vi "ReactionWheel RT - autostarted.vi"() -> ()   [LabVIEW 2021]
uses:
  <vilib>/Platform/TimedLoop/XDataNode/timing_clust.ctl
  <vilib>/Platform/TimedLoop/XDataNode/nitl_modes.ctl
  <vilib>/Platform/TimedLoop/XDataNode/wakeup.ctl
  <vilib>/myRIO/Instrument Drivers/Onboard IO/UART/typedef/VISA Configuration.ctl
  <vilib>/myRIO/Instrument Drivers/Onboard IO/DIO/typedefs/DIO Reference.ctl
  <vilib>/myRIO/Common/Instrument Driver Framework/Utilities/typedefs/myRIO Generic Hardware Reference.ctl
  <vilib>/myRIO/Common/Instrument Driver Framework/Utilities/typedefs/Hardware Version Enum.ctl
  <vilib>/myRIO/Common/Instrument Driver Framework/Utilities/typedefs/myRIO v1.0 Reference.ctl
  <vilib>/myRIO/Common/Instrument Driver Framework/Utilities/typedefs/Generic FPGA Reference.ctl
  <vilib>/myRIO/Common/Instrument Driver Framework/myRIO v1.0/DIO/typedefs/DIO Channels List.ctl
  <vilib>/myRIO/Common/Instrument Driver Framework/myRIO v1.0/DIO/typedefs/DIO Channels Enum.ctl
  <vilib>/userdefined/High Color/nirio_resource_hc.ctl
  <vilib>/myRIO/Instrument Drivers/Onboard IO/PWM/typedefs/PWM Reference.ctl
  <vilib>/myRIO/Common/Instrument Driver Framework/myRIO v1.0/PWM/typedefs/PWM Channels Enum.ctl
  <vilib>/myRIO/Instrument Drivers/Onboard IO/PWM/typedefs/PWM Configuration.ctl
  <vilib>/myRIO/Common/Instrument Driver Framework/Utilities/vis/Is FPGA Ref Available.vi
  <vilib>/myRIO/Common/Instrument Driver Framework/myRIO v1.0/PWM/vis/myRIO v1.1 Open PWM.vi
  <vilib>/myRIO/Instrument Drivers/Onboard IO/PWM/vis/Set Duty Cycle and Frequency.vi
  <vilib>/myRIO/Common/Instrument Driver Framework/myRIO v1.0/DIO/vis/myRIO v1.1 Open DIO.vi
  <vilib>/myRIO/Instrument Drivers/Onboard IO/DIO/vis/Write.vi
  <vilib>/myRIO/Common/Instrument Driver Framework/Utilities/vis/Validate Channels.vi
  <vilib>/myRIO/Common/Instrument Driver Framework/myRIO v1.0/PWM/vis/myRIO v1.0 Reserve PWM.vi
  <vilib>/myRIO/Common/Instrument Driver Framework/myRIO v1.0/DIO/vis/myRIO v1.0 Reserve DIO.vi
  <vilib>/myRIO/Common/Instrument Driver Framework/myRIO v1.0/PWM/vis/myRIO v1.0 Build MUX Configuration PWM.vi
  <vilib>/myRIO/Common/Instrument Driver Framework/myRIO v1.0/Resource Manager/vis/myRIO v1.0 Reserve Channel List.vi
  <vilib>/myRIO/Common/Instrument Driver Framework/myRIO v1.0/DIO/vis/myRIO v1.0 Build MUX Configuration DIO.vi
  <vilib>/myRIO/Common/Instrument Driver Framework/myRIO v1.0/Resource Manager/vis/myRIO v1.0 Create Configuration List.vi
  <vilib>/myRIO/Common/Instrument Driver Framework/myRIO v1.0/Resource Manager/vis/myRIO v1.0 Reserve Channel.vi
  <vilib>/myRIO/Common/Instrument Driver Framework/myRIO v1.0/Resource Manager/vis/myRIO v1.0 Unreserve Channel.vi
  <vilib>/myRIO/Common/Instrument Driver Framework/myRIO v1.0/Resource Manager/vis/myRIO v1.0 Build Mutex Name.vi
  <vilib>/Instr/_visa.llb/VISA Configure Serial Port (Instr).vi
  <vilib>/Utility/VariantDataType/GetNumericInfo.vi
  <vilib>/Utility/error.llb/Error Cluster From Error Code.vi
  <vilib>/myRIO/Common/Instrument Driver Framework/myRIO v1.0/myRIO v1.1 Open.vi
  <vilib>/myRIO/Common/Instrument Driver Framework/Utilities/vis/IO Manager.vi
  <vilib>/myRIO/Common/Instrument Driver Framework/Utilities/vis/Configuration Manager.vi
  <vilib>/myRIO/Common/Instrument Driver Framework/myRIO v1.0/Resource Manager/vis/myRIO v1.0 Configure IO.vi
  <vilib>/myRIO/Common/Instrument Driver Framework/myRIO v1.0/myRIO v1.0 Close.vi
  <vilib>/myRIO/Common/Instrument Driver Framework/myRIO v1.0/PWM/vis/myRIO v1.0 Write PWM.vi
  <vilib>/myRIO/Common/Instrument Driver Framework/myRIO v1.0/DIO/vis/myRIO v1.0 Write DIO.vi
  <vilib>/addons/control/pid/pid.llb/PID (DBL).vi
  <vilib>/platform/TimedLoop/XDataNode/XDataNode.xnode
  <vilib>/myRIO/Express VI/Onboard IO/UART/UART Express VI.xnode
  <vilib>/myRIO/Express VI/Onboard IO/PWM/PWM Express VI.xnode
  <vilib>/myRIO/Instrument Drivers/Onboard IO/PWM/vis/myRIO PWM Open.xnode
  <vilib>/myRIO/Express VI/Onboard Devices/LED/LED Express VI.xnode
  <vilib>/myRIO/Instrument Drivers/Onboard IO/DIO/vis/myRIO DIO Open.xnode
  <vilib>/myRIO/Instrument Drivers/Onboard IO/UART/UART.lvlib
  <vilib>/myRIO/Instrument Drivers/Onboard IO/PWM/PWM.lvlib
  <vilib>/addons/control/pid/NI_PID_pid.lvlib
  <vilib>/Platform/TimedLoop/XDataNode/XDNodeRunTimeDep.lvlib
  <vilib>/myRIO/Instrument Drivers/Onboard IO/DIO/DIO.lvlib
panel:
  in  "Deadzone off/on":bool
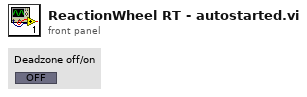
[diagram p1: front panel]
types:
  T1 = typedef "PWM.lvlib/PWM Reference.ctl" = cluster{"myRIO Reference":T2, "PWM Channels Enum":T6, "PWM Configuration":T7}
  T2 = typedef "myRIO Generic Hardware Reference.ctl" = cluster{"myRIO Model":T3, "myRIO Hardware Reference":T4}
  T3 = typedef "Hardware Version Enum.ctl" = enum16{"Unknown", "myRIO-1900", "myRIO-1950", "roboRIO", "NI ELVIS RIO CM", "ELVIS III"}
  T4 = typedef "myRIO v1.0 Reference.ctl" = cluster{"Generic FPGA Reference":T5, "Allow multiple opens":bool}
  T5 = typedef "Generic FPGA Reference.ctl" = refnum<k20>
  T6 = typedef "PWM Channels Enum.ctl" = enum16{"Not Connected", "C/PWM0", "C/PWM1", "A/PWM0", "A/PWM1", "A/PWM2", "A/PWM3", "A/PWM4", "A/PWM5", "A/PWM6", "A/PWM7", "A/PWM8", "A/PWM9", "A/PWM10", "A/PWM11", "A/PWM12", "A/PWM13", "A/PWM14", "A/PWM15", "A/PWM16", "A/PWM17", "A/PWM18", "A/PWM19", "B/PWM0", "B/PWM1", "B/PWM2", "B/PWM3", "B/PWM4", "B/PWM5", "B/PWM6", "B/PWM7", "B/PWM8", "B/PWM9", "B/PWM10", "B/PWM11", "B/PWM12", "B/PWM13", "B/PWM14", "B/PWM15", "B/PWM16", "B/PWM17", "B/PWM18", "B/PWM19", "PWM/PWM0", "PWM/PWM1", "PWM/PWM2", "PWM/PWM3", "PWM/PWM4", "PWM/PWM5", "PWM/PWM6", "PWM/PWM7", "PWM/PWM8", "PWM/PWM9"}
  T7 = typedef "PWM.lvlib/PWM Configuration.ctl" = cluster{"Frequency":dbl, "Duty Cycle":dbl}
  T8 = typedef "nirio_resource_hc.ctl" = tag
  T9 = typedef "UART.lvlib/VISA Configuration.ctl" = cluster{"baud rate (9600)":u32, "data bits (8)":u16, "parity (0:none)":enum16{"None", "Odd", "Even", "Mark", "Space"}, "stop bits (10: 1 bit)":u16, "flow control (0:none)":u16, "termination char\n(0xA = '\\n' = LF) ":u8, "Enable Termination\nChar (T)":bool, "timeout (10sec)":u32}
  T10 = typedef "DIO.lvlib/DIO Reference.ctl" = cluster{"myRIO Reference":T2, "DIO Channels List":T11}
  T11 = typedef "DIO Channels List.ctl" = T12[]
  T12 = typedef "DIO Channels Enum.ctl" = enum16{"Not Connected", "C/DIO0", "C/DIO1", "C/DIO2", "C/DIO3", "C/DIO4", "C/DIO5", "C/DIO6", "C/DIO7", "A/DIO0", "A/DIO1", "A/DIO2", "A/DIO3", "A/DIO4", "A/DIO5", "A/DIO6", "A/DIO7", "A/DIO8", "A/DIO9", "A/DIO10", "A/DIO11", "A/DIO12", "A/DIO13", "A/DIO14", "A/DIO15", "A/DIO16", "A/DIO17", "A/DIO18", "A/DIO19", "B/DIO0", "B/DIO1", "B/DIO2", "B/DIO3", "B/DIO4", "B/DIO5", "B/DIO6", "B/DIO7", "B/DIO8", "B/DIO9", "B/DIO10", "B/DIO11", "B/DIO12", "B/DIO13", "B/DIO14", "B/DIO15", "B/DIO16", "B/DIO17", "B/DIO18", "B/DIO19", "LED0", "LED1", "LED2", "LED3", "Button0", "DIO/DIO0", "DIO/DIO1", "DIO/DIO2", "DIO/DIO3", "DIO/DIO4", "DIO/DIO5", "DIO/DIO6", "DIO/DIO7", "DIO/DIO8", "DIO/DIO9", "SPI/CS0", "SPI/CS1", "SPI/CS2", "SPI/CS3", "LED RADIO (Green)", "LED RADIO (Red)", "LED COMM (Green)", "LED COMM (Red)", "LED MODE (Green)", "LED MODE (Red)"}
  T13 = typedef "XDNodeRunTimeDep.lvlib/timing_clust.ctl" = cluster{"Expected End [f-1]":u64, "Actual End [f-1]":u64, "Finished Late? [f-1]":bool, "Expected End [i-1]":u64, "Actual End [i-1]":u64, "Finished Late? [i-1]":bool, "Expected Start [i]":u64, "Actual Start [i]":u64, "Expected Start [f]":u64, "Actual Start [f]":u64, "Source Name":string, "Structure Name":string, "Period":i64, "Deadline":i64, "Offset":i64, "Start":i64, "Priority":i32, "Timeout":i32, "Mode":T14, "Wakeup Reason":T15, "Error":errorcluster, "Source Type":string, "Secondary Source Type":string, "Global End Time":u64, "Global Start Time":u64, "Frame Duration":u64, "Iteration Duration":u64, "Assigned CPU":i32, "I/O Scan Engine Mode":u32}
  T14 = typedef "XDNodeRunTimeDep.lvlib/nitl_modes.ctl" = enum32{"No Change", "Process missed periods, maintain original phase", "Discard missed periods, maintain original phase", "Process missed periods, ignore original phase", "Discard missed periods, ignore original phase"}
  T15 = typedef "XDNodeRunTimeDep.lvlib/wakeup.ctl" = enum32{"Normal", "Aborted", "Asynchronous wakeup", "Timing source error", "Timed loop error", "Timeout"}
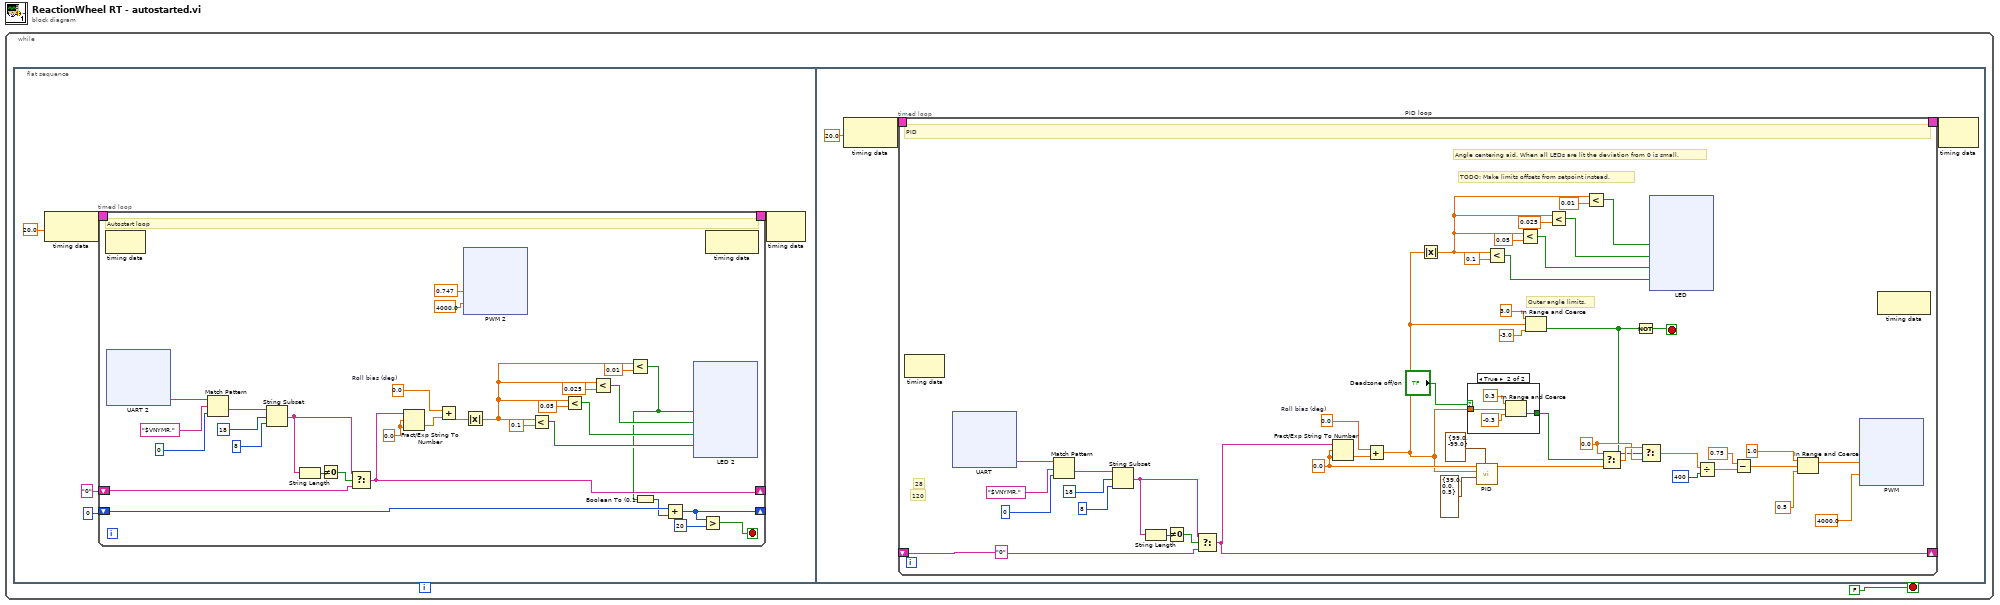
[diagram p0: block diagram]
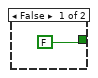
[diagram p2: hidden frame]
diagram:
  n1 = while {
    stop <- FALSE stop-if-true
    n2 = flat-sequence {
      frame #0 {
        n3 = node-c288(20.0 ("UART read period (ms)")) -> (w6:T13)
        n4 = timed-loop {
          timing: w6 -> [_]
          timing-out: [_] -> w5
          shift-right: [w18] -> _
          shift-left: "0" -> [w19]
          shift-right: [w9] -> _
          shift-left: 0 -> [w11]
          stop <- w8 stop-if-true
          w16 = 0.0  # Roll bias (deg)
          w23 = 0.0
          # "Autostart loop"
          n5 = node-c288() -> ()  [unwired: 1 in, 1 out]
          n6 = xnode "UART 2"() -> ("Characters Read"=w29:string)  [unwired: 1 in, 1 out]
          n7 = Match Pattern(string=w29, regular expression="$VNYMR,", offset (0)=0) -> (after substring=w28:string)  [unwired: 3 out]
          n8 = String Subset(string=w28, offset (0)=18, length (rest)=8) -> (substring=w20:string)
          n9 = String Length(string=w20) -> (length=w22:i32)
          n10 = Not Equal To 0?(x=w22) -> (x != 0?=w21:bool)
          n11 = Select(t=w20, s=w21, f=w19) -> (s? t:f=w18:string)
          n12 = Fract/Exp String To Number(string=w18, offset=w23, default (0 dbl)=w23) -> (number=w15:dbl)  [unwired: 1 in, 1 out]
          n13 = Add(x=w16, y=w15) -> (x+y=w17:dbl)
          n14 = xnode "PWM 2"("Duty Cycle"=0.747, "Frequency [Hz]"=4000.0 ("PWMfrekvens")) -> ()  [unwired: 1 in, 1 out]
          n15 = Absolute Value(x=w17) -> (abs(x)=w30:dbl)
          n16 = Less?(x=w30, y=0.1) -> (x < y?=w37:bool)
          n17 = Less?(x=w30, y=0.05) -> (x < y?=w34:bool)
          n18 = Less?(x=w30, y=0.025) -> (x < y?=w32:bool)
          n19 = Less?(x=w30, y=0.01) -> (x < y?=w12:bool)
          n20 = Boolean To (0,1)(Boolean=w12) -> (0, 1=w10:i16)
          n21 = Add(x=w11, y=w10) -> (x+y=w9:i32)
          n22 = xnode "LED 2"("LED0"=w12, "LED1"=w32, "LED2"=w34, "LED3"=w37) -> ()  [unwired: 1 in, 1 out]
          n23 = Greater?(x=w9, y=20) -> (0:w8:bool)
          n24 = node-c288() -> ()  [unwired: 1 in, 1 out]
        }
        n25 = node-c288(w5) -> ()  [unwired: 1 out]
      }
      frame #1 {
        n26 = node-c288(20.0 ("UART read period (ms)")) -> (w137:T13)
        n27 = timed-loop "PID loop" {
          timing: w137 -> [_]
          timing-out: [_] -> w136
          shift-right: [w158] -> _
          shift-left: "0" -> [w159]
          stop <- w138 stop-if-true
          w150 = 0.0
          w174 = 0.0  # Roll bias (deg)
          w165 = 0.0
          # "TODO: Make limits offsets from setpoint instead."
          # "Angle centering aid. When all LEDs are lit the deviation from 0 is small."
          # "Outer angle limits."
          # "28"
          # "120"
          # "PID"
          n28 = node-c288() -> ()  [unwired: 1 in, 1 out]
          n29 = xnode "UART"() -> ("Characters Read"=w181:string)  [unwired: 1 in, 1 out]
          n30 = Match Pattern(string=w181, regular expression="$VNYMR,", offset (0)=0) -> (after substring=w180:string)  [unwired: 3 out]
          n31 = String Subset(string=w180, offset (0)=18, length (rest)=8) -> (substring=w160:string)
          n32 = String Length(string=w160) -> (length=w162:i32)
          n33 = Not Equal To 0?(x=w162) -> (x != 0?=w161:bool)
          n34 = Select(t=w160, s=w161, f=w159) -> (s? t:f=w158:string)
          n35 = Fract/Exp String To Number(string=w158, offset=w165, default (0 dbl)=w165) -> (number=w175:dbl)  [unwired: 1 in, 1 out]
          n36 = Add(x=w174, y=w175) -> (x+y=w143:dbl)
          n37 = Absolute Value(x=w143) -> (abs(x)=w140:dbl)
          n38 = case shown="True" "Deadzone off/on" {
            tunnel: [FALSE w224] -> w156
            tunnel: w143 -> [_ w223]
            frame False {
            }
            frame True {
              n39 = In Range and Coerce(upper limit=0.3 ("Angle deadzone upper limit"), x=w223, lower limit=-0.3 ("Angle deadzone lower limit")) -> (In Range?=w224:bool)  [unwired: 1 out]
            }
          }
          n40 = call-poly <vilib>:"PID.vi"("output range"=cluster{"Maximum":dbl, "Minimum":dbl} {"Maximum"=99.0, "Minimum"=-99.0} ("PID output range"), "PID gains"=cluster{"P":dbl, "I":dbl, "D":dbl} {"P"=39.0, "I"=0.0, "D"=0.5}, "process variable"=w143, "setpoint"=w165) -> ("output"=w157:dbl)  [unwired: 6 in, 1 out]
          n41 = Less?(x=w140, y=0.1) -> (x < y?=w149:bool)
          n42 = Less?(x=w140, y=0.05) -> (x < y?=w146:bool)
          n43 = In Range and Coerce(upper limit=3.0 ("Angle deadzone upper limit"), x=w143, lower limit=-3.0 ("Angle deadzone lower limit")) -> (In Range?=w139:bool)  [unwired: 1 out]
          n44 = Less?(x=w140, y=0.025) -> (x < y?=w144:bool)
          n45 = Less?(x=w140, y=0.01) -> (x < y?=w141:bool)
          n46 = Select(t=w150, s=w156, f=w157) -> (s? t:f=w151:dbl)
          n47 = Not(x=w139) -> (.not. x?=w138:bool)
          n48 = Select(t=w151, s=w139, f=w150) -> (s? t:f=w152:dbl)
          n49 = xnode "LED"("LED0"=w141, "LED1"=w144, "LED2"=w146, "LED3"=w149) -> ()  [unwired: 1 in, 1 out]
          n50 = Divide(x=w152, y=400) -> (x/y=w166:dbl)
          n51 = Subtract(x=0.75, y=w166) -> (x-y=w171:dbl)
          n52 = In Range and Coerce(upper limit=1.0 ("Max PWM"), x=w171, lower limit=0.5 ("Min PWM")) -> (coerced(x)=w172:dbl)  [unwired: 1 out]
          n53 = xnode "PWM"("Duty Cycle"=w172, "Frequency [Hz]"=4000.0 ("PWMfrekvens")) -> ()  [unwired: 1 in, 1 out]
          n54 = node-c288() -> ()  [unwired: 1 in, 1 out]
        }
        n55 = node-c288(w136) -> ()  [unwired: 1 out]
      }
    }
  }
